vi "enumerateStaticDependencies.vi"(8 "error in (no error)":errorcluster, 11 "MeasurementSMO":refnum<class "MeasurementSMO.lvclass">) -> (0 "error out":errorcluster, 2 "Static Dependencies":refnum<class "Dependency.lvclass">[](array[class]), 3 "MeasurementSMO out":refnum<class "MeasurementSMO.lvclass">)   [LabVIEW 2020, in "MeasurementSMO.lvclass"]
uses:
  MeasurementSMO.lvclass
  <vilib>/JKI/JKI SMO/Dependency/Dependency.lvclass
  <vilib>/JKI/JKI SMO/SMO/SMO.lvclass
panel:
  # "For instructions on how to use the JKI State Machine Objects, examples and video tutorials, visit:\nhttp://jki.net/state-machine-objects/\n\nJKI State Machine Objects™\nhttp://jki.net/state-machine-objects/\nCopyright (C) 2005-2015, JKI <info@jki.net>\nALL RIGHTS RESERVED"
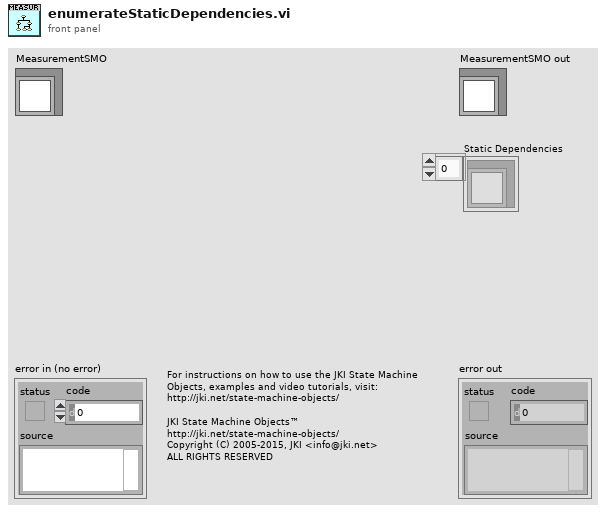
[diagram p1: front panel]
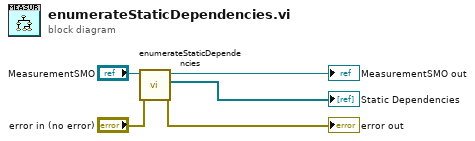
[diagram p0: block diagram]
diagram:
  n1 = call-parent "enumerateStaticDependencies.vi"("error in (no error)"="error in (no error)", "SMO"="MeasurementSMO") -> ("error out"=→"error out":errorcluster, "Static Dependencies"=→"Static Dependencies":refnum<class "Dependency.lvclass">[], "SMO out"=→"MeasurementSMO out":refnum<class "MeasurementSMO.lvclass">)  [unwired: 7 in]
